vi "ChooseOne.vi"(8 "False Code":string, 9 "Comparison":string(combo)="True", 10 "True Code":string, 11 "Data In":T1) -> (2 "Data Out":T1={"Port"="", "All Code"="Hi"})   [LabVIEW 2016]
uses:
  uPythonX/PythonData.ctl
  uPythonX/uPythonX.xctl
panel:
  out "resulting string":string
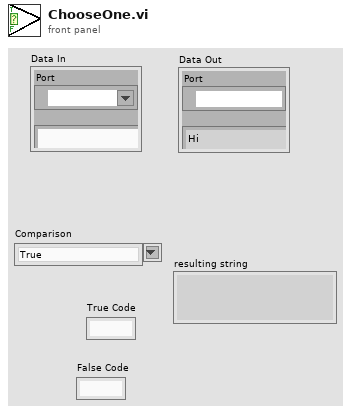
[diagram p1: front panel]
types:
  T1 = typedef "uPythonX.xctl/PythonData.ctl" = cluster{"Port":refnum<visa-resource-name>, "All Code":string}
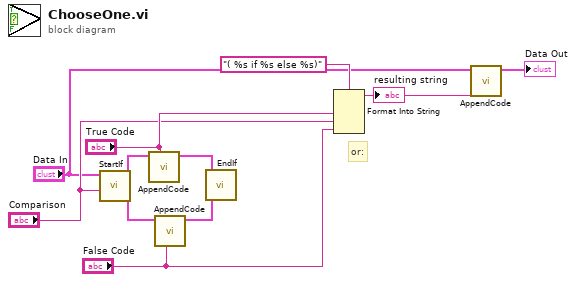
[diagram p0: block diagram]
diagram:
  # "or:"
  n1 = call "StartIf.vi"("Comparison"="Comparison", "Data In"="Data In") -> ("False Out"=w9:T1, "True Out"=w11:T1)  [unwired: 8 in]
  n2 = call "AppendCode.vi"("New Code"="True Code", "Data In"=w11) -> ("Data Out"=w10:T1)  [unwired: 9 in]
  n3 = call "AppendCode.vi"("New Code"="False Code", "Data In"=w9) -> ("Data Out"=w8:T1)  [unwired: 9 in]
  n4 = call "EndIf.vi"("False In"=w8, "True In"=w10) -> ()  [unwired: 9 in, 1 out]
  n5 = Format Into String(format string="( %s if %s else %s)", "True Code", "Comparison", "False Code") -> (resulting string=w1:string)  [unwired: 2 in, 1 out]
  "resulting string" <- w1
  n6 = call "AppendCode.vi"("New Code"=w1, "Data In"="Data In") -> ("Data Out"=→"Data Out":T1)  [unwired: 9 in]
